vi "Get Self Queue Alias.vi"(11 "Addresses in":refnum<class "Addresses.lvclass">) -> (2 "Self Queue Alias":string)   [LabVIEW 2021, in "jettl.lvlib" / "Addresses.lvlib" / "Addresses.lvclass"]
uses:
  Addresses.lvclass
  Addresses.lvclass/Addresses.ctl
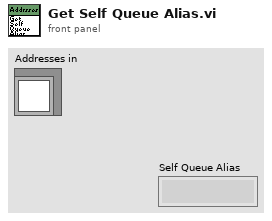
[diagram p1: front panel]
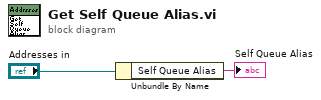
[diagram p0: block diagram]
diagram:
  n1 = Unbundle By Name("Addresses in") -> ("Self Queue Alias"=→"Self Queue Alias":string)
